vi "sendcmd.vi"(1 "error in (no error)":errorcluster, 2 "parameter":string, 3 "command in":string) -> (0 "error out":errorcluster)   [LabVIEW 2017]
doc: "Sends the command with parameter to the Cornerstone"
uses:
  m_globals.vi
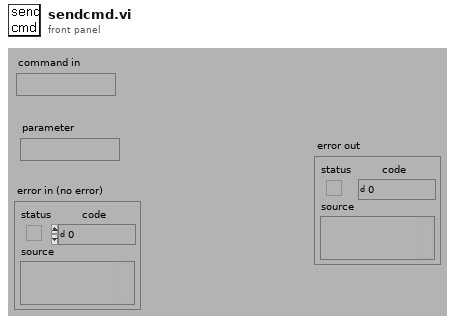
[diagram p1: front panel]
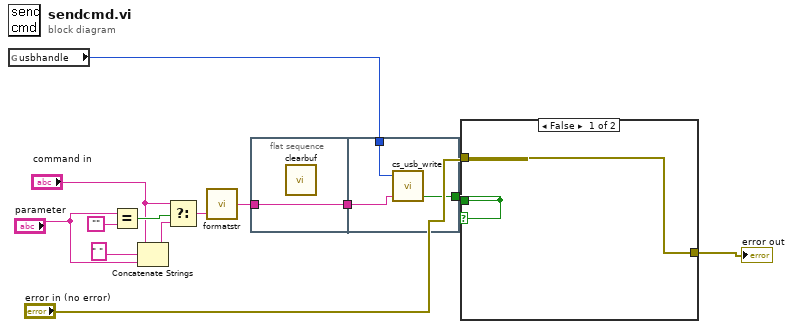
[diagram p0: block diagram]
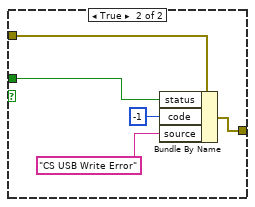
[diagram p2: hidden frame]
diagram:
  n1 = global read "m_globals.vi" "usbhandle"() -> (w6:i32)
  n2 = Equal?(x="parameter", y="") -> (x = y?=w10:bool)
  n3 = Concatenate Strings("command in", " ", "parameter") -> (w8:string)
  n4 = Select(t="command in", s=w10, f=w8) -> (s? t:f=w7:string)
  n5 = call "formatstr.vi"("command in"=w7) -> ("Formated command string"=w5:string)
  n6 = flat-sequence {
    tunnel: w5 -> [w14]
    tunnel: [w14] -> w1
    tunnel: w6 -> [w17]
    tunnel: [w15] -> w2
    tunnel: w1 -> [w16]
    frame #0 {
      n7 = call "clearbuf.vi"() -> ()  [unwired: 1 in, 1 out]
    }
    frame #1 {
      n8 = call "cs_usb_write.vi"("string to send"=w16, "handle"=w17) -> ("Error"=w15:bool)  [unwired: 3 in]
    }
  }
  n9 = case shown="False" w2 {
    tunnel: "error in (no error)" -> [w18 w20]
    tunnel: [w18 w21] -> w3
    tunnel: w2 -> [_ w23]
    frame False {
    }
    frame True {
      n10 = Bundle By Name(cluster=w20, "status"=w23, "code"=-1, "source"="CS USB Write Error") -> (w21:errorcluster)
    }
  }
  "error out" <- w3
